vi "final_control_mk12_061625.vi"() -> ()   [LabVIEW 2023]
doc: "Simplified example program for initializing the COM port, determining the data frame of up to 26 Alicats, acquiring the data of the same number of Alicats, displaying the data of the one with the selected unit ID, and writing a setpoint to the same selected unit ID.\n\nThis is a slightly more feature rich version of the Alicat Simplified Driver Example, and contains an example of a method for interfacing with up to 26 Alicats on a single COM port by means of for loops with shift registers to handle sequential commands to each included Alicat. This also contains a method to write a setpoint to the same selected unit.\n\nIf coding for multiple Alicats on a single COM port without the use of for loops with shift registers, ensure that each Alicat command is executed sequentially. Alicat's RS-232/485 does not work if multiple devices are responding simultaneously."
uses:
  <vilib>/Platform/TimedLoop/XDataNode/timing_clust.ctl
  <vilib>/Platform/TimedLoop/XDataNode/nitl_modes.ctl
  <vilib>/Platform/TimedLoop/XDataNode/wakeup.ctl
  <vilib>/DAQmx/write.llb/DAQmx Write (Analog 1D DBL NChan 1Samp).vi
  <vilib>/DAQmx/read.llb/DAQmx Read (Analog DBL 1Chan 1Samp).vi
  <extravilib>/ChannelInstances/Tag-bool/Read With Abort.vi
  <extravilib>/ChannelInstances/Tag-bool/Write With Abort.vi
  <vilib>/Utility/file.llb/Write Delimited Spreadsheet (string).vi
  <extravilib>/ChannelInstances/Tag-bool/Instantiate.vi
  <vilib>/Utility/file.llb/Read Delimited Spreadsheet (DBL).vi
  <extravilib>/ChannelInstances/Tag-bool/EndpointRead.vi
  <vilib>/DAQmx/miscellaneous.llb/DAQmx Fill In Error Info.vi
  <extravilib>/ChannelInstances/Tag-bool/Endpoint.vi
  <vilib>/platform/TimedLoop/XDataNode/XDataNode.xnode
  <vilib>/express/express arith-compare/Formula/XNode/ExpressFormulaBlockNode.xnode
  <vilib>/Platform/TimedLoop/XDataNode/XDNodeRunTimeDep.lvlib
  <extravilib>/ChannelInstances/Tag-bool.lvlib
panel:
  in  "Tab Control":enum32{"Page 1", "Page 2"}(tab)
  in  "COM Port Settings":T1={"Baud Rate"=enum."19200", "VISA Sesssion In"="MassFlowControllers"}
  out "Range Exceeded":bool
  out "Error Present":bool
  out "Error Text":string
  out "Elapsed Time [ms]\n(all units)":dbl caption="Elapsed Time (s)"
  in  "Minimum time between \nreadings [ms] (all units)":u32
  in  "Device ID's \nto Include:":T2={"A"=TRUE, "B"=TRUE, "C"=TRUE, "D"=TRUE, "E"=TRUE, "F"=TRUE, "G"=FALSE, "H"=FALSE, "I"=FALSE, "J"=FALSE, "K"=FALSE, "L"=FALSE, "M"=FALSE, "N"=FALSE, "O"=FALSE, "P"=FALSE, "Q"=FALSE, "R"=FALSE, "S"=FALSE, "T"=FALSE, "U"=FALSE, "V"=FALSE, "W"=FALSE, "X"=FALSE, "Y"=FALSE, "Z"=FALSE}
  out "Active Device":u16(ring) items=["A", "B", "C", "D", "E", "F"]
  out "Meas. Data (for active device)":T3
  in  "Write File":path
  in  "Hold Time\n[min]":dbl=16.0 min=17.0
  out "N":i32
  in  "Read File":path
  in  "End Program":bool
  in  "Start From:":i32=1
  in  "t_read [ms]":dbl=24000.0
  out "T_SCh [C]":dbl format="%0.2f"
  out "iter start":string
  out "Iter_Duration [ms]":string
  out "C_CH4 [ppm]":string
  out "C_H2 [ppm]":string
  in  "Start Times":path
  in  "API Key":string="V1WFARF28XTM5DW7"
  in  "Send Alerts?":bool=TRUE
  out "C_H2S [ppm]":string
  out "len_SP":i32
  out "Setpoints":dbl[][](array[numeric])=[[4.2, 3.3], [69.0, 4.2]]
  out "Z":dbl[](array[numeric])
  out "ASP":dbl
  out "BSP":dbl
  out "CSP":dbl
  out "DSP":dbl
  out "ESP":dbl
  out "FSP":dbl
  out "N_read":i32
  out "Iter_#":string
  out "V_D":string
  out "V_H":string
  out "all rows":dbl[][](array[numeric])
  out "T_SCh":string
  out "Iteration Duration":i64
  out "read_cnt_true":i32
  out "iter_dur_read [ms]":i64
  out "t_diff":dbl
  out "date":string
  out "time":string
  # "Totalizer Timer"
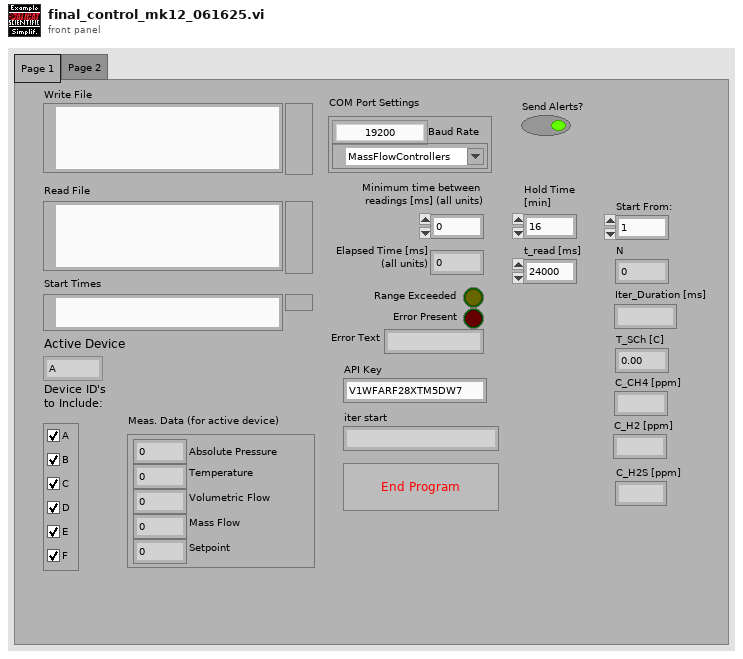
[diagram p1: front panel]
types:
  T1 = cluster{"Baud Rate":enum8{"2400", "9600", "19200", "38400", "57600", "115200", "Unknown"}, "VISA Sesssion In":refnum<visa-resource-name>}
  T2 = cluster{"A":bool, "B":bool, "C":bool, "D":bool, "E":bool, "F":bool, "G":bool, "H":bool, "I":bool, "J":bool, "K":bool, "L":bool, "M":bool, "N":bool, "O":bool, "P":bool, "Q":bool, "R":bool, "S":bool, "T":bool, "U":bool, "V":bool, "W":bool, "X":bool, "Y":bool, "Z":bool}
  T3 = cluster{"Absolute Pressure":dbl, "Gauge/Diff. Pressure":dbl, "Barometric Pressure":dbl, "Temperature":dbl, "Volumetric Flow":dbl, "Mass Flow":dbl, "Setpoint":dbl, "Valve Drive":dbl, "Totalizer":dbl, "[hr]":dbl, "[min]":dbl, "[sec]":dbl, "Totalizer Average Flow":dbl, "Totalizer Peak Flow":dbl, "Gas selected":string}
  T4 = cluster{"Unit ID":string, "Baud Rate":enum8{"2400", "9600", "19200", "38400", "57600", "115200", "Unknown"}, "VISA Sesssion In":refnum<visa-resource-name>}
  T5 = enum16{"Request Ack", "Set Setpoint", "Set Lo Limit", "Set Hi Limit", "Set Prop Band 0-99.9", "Set Integral 0-9.99", "Set Derivative 0-5.0", "Read Int Temp", "Read Ext Temp", "Read Setpoint", "Read Low Limit", "Read High Limit", "Read Prop Band", "Read Integral", "Read Derivative "}
  T6 = typedef "XDNodeRunTimeDep.lvlib/timing_clust.ctl" = cluster{"Expected End [f-1]":u64, "Actual End [f-1]":u64, "Finished Late? [f-1]":bool, "Expected End [i-1]":u64, "Actual End [i-1]":u64, "Finished Late? [i-1]":bool, "Expected Start [i]":u64, "Actual Start [i]":u64, "Expected Start [f]":u64, "Actual Start [f]":u64, "Source Name":string, "Structure Name":string, "Period":i64, "Deadline":i64, "Offset":i64, "Start":i64, "Priority":i32, "Timeout":i32, "Mode":T7, "Wakeup Reason":T8, "Error":errorcluster, "Source Type":string, "Secondary Source Type":string, "Global End Time":u64, "Global Start Time":u64, "Frame Duration":u64, "Iteration Duration":u64, "Assigned CPU":i32, "I/O Scan Engine Mode":u32}
  T7 = typedef "XDNodeRunTimeDep.lvlib/nitl_modes.ctl" = enum32{"No Change", "Process missed periods, maintain original phase", "Discard missed periods, maintain original phase", "Process missed periods, ignore original phase", "Discard missed periods, ignore original phase"}
  T8 = typedef "XDNodeRunTimeDep.lvlib/wakeup.ctl" = enum32{"Normal", "Aborted", "Asynchronous wakeup", "Timing source error", "Timed loop error", "Timeout"}
  T9 = typedef "Tag-bool.lvlib/))Channel.ctl" = refnum<queue>
  T10 = enum8{"2400", "9600", "19200", "38400", "57600", "115200", "Unknown"}
  T11 = cluster{"Absolute Pressure":bool, "Gauge/Diff. Pressure":bool, "Barometric Pressure":bool, "Temperature":bool, "Volumetric":bool, "Mass":bool, "Setpoint":bool, "Valve Drive":bool, "Totalizer":bool, "Totalizer Timer":bool, "Totalizer Average Flow":bool, "Totalizer Peak Flow":bool, "Gas Selected":bool, "Tot. Timer Format":u16}
  T12 = cluster{"Controller Full Scale":dbl, "Controller Select":u16, "Control Range":enum16{"Normal", "Inverted", "Bidirectional", "Unknown"}}
  T13 = cluster{"Controller Full Scale":dbl, "Controller Select":u16, "Control Range":enum16{"Normal", "Inverted", "Bidirectional", "Unknown"}}[]
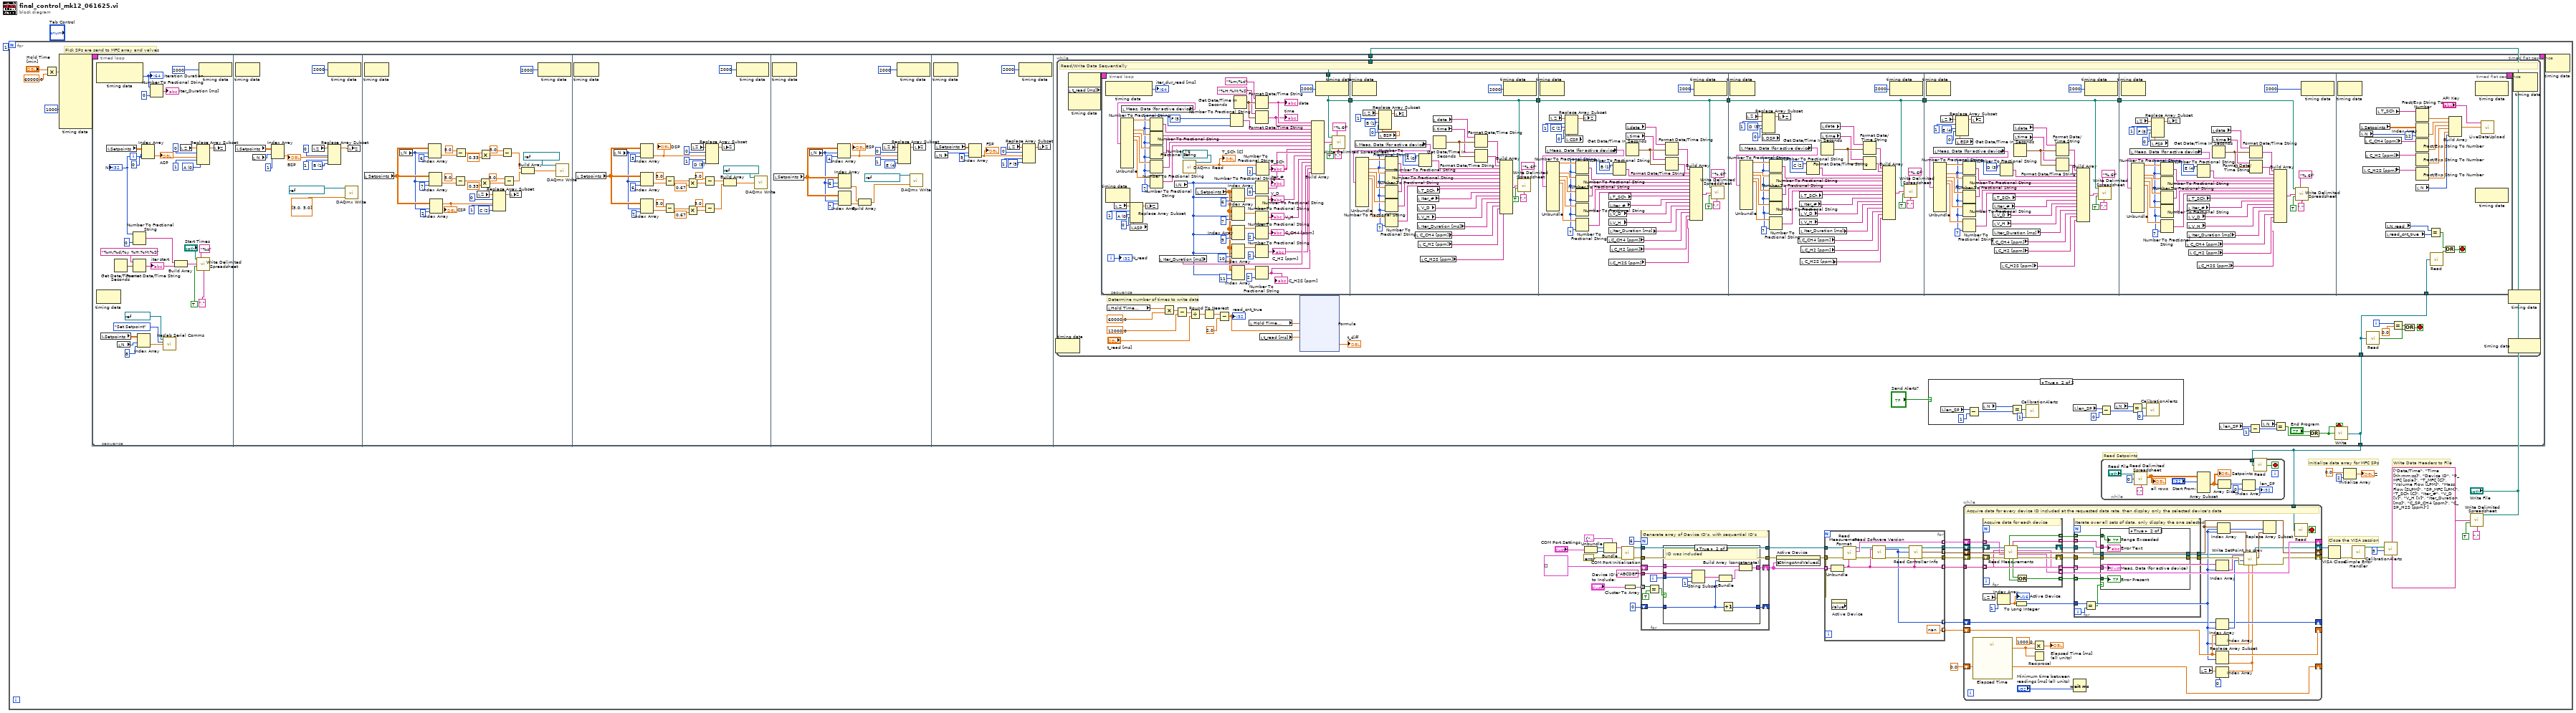
[diagram p0: block diagram]
diagram:
  n1 = for {
    N: 1 -> [_]
    # "Pick SPs are send to MFC array and valves"
    # "Write Data Headers to File"
    # "Read Setpoints"
    # "Initialize data array for MFC SPs"
    # "Close the VISA session"
    n2 = Multiply(x="Hold Time\n[min]", y=60000.0) -> (x*y=w5:dbl)
    n3 = node-c288(w5, i64 1000 ("Offset")) -> (w46:T6)  [unwired: 8 in]
    n4 = timed-loop "Write Data" {
      timing: w46 -> [_]
      timing-out: [_] -> w45
      tunnel: [w59] -> w12
      tunnel: "Write File" -> [w58]
      i -> [w73]
      stop <- w216 stop-if-true
      n5 = timed-sequence {
        timing: _ -> [_]
        timing-out: _ -> [_]
        tunnel: [w61] -> w59
        tunnel: w58 -> [w60]
        n6 = timed-flat-sequence {
          tunnel: [w211] -> w61
          tunnel: w60 -> [w212]
          frame #0 {
            w83 = u16 0 items=["A", "B", "C", "D", "E", "F"]
            n7 = node-c288() -> (w77:i64)  [unwired: 1 in, 1 out]
            "Iteration Duration" <- w77
            n8 = local read "Setpoints"() -> (w67:dbl[][])
            n9 = local read "Setpoints"() -> (w90:dbl[][])
            n10 = Get Date/Time In Seconds() -> (seconds since 1Jan1904=w78:timestamp)
            n11 = local read "N"() -> (w66:i32)
            n12 = Number To Fractional String(number=w73, precision (6)=i16 0) -> (F-format string=w71:string)  [unwired: 2 in]
            n13 = Format Date/Time String(time format string (%c)="%m/%d/%y %H:%M:%S", seconds (now)=w78) -> (date/time string=w70:string)  [unwired: 1 in]
            "iter start" <- w70
            n14 = Index Array(array=w67, index (row)=w66, index (col)=8 ("disabled index (col)")) -> (element=w64:dbl)
            n15 = Index Array(array=w90, index (row)=w73, index (col)=0 ("index (row)")) -> (element=w88:dbl)
            "ASP" <- w88
            n16 = Number To Fractional String(number=w77, precision (6)=i16 0) -> (F-format string=→"Iter_Duration [ms]":string)  [unwired: 2 in]
            n17 = call "Neslab Serial Comms.vi"("VISA resource name"=refnum<visa-resource-name> "COM1", "Command"=T5."Set Setpoint", "Set Value"=w64) -> ()  [unwired: 6 in, 7 out]
            n18 = Build Array(w71, w70) -> (w69:string[])
            n19 = local read "Z"() -> (w86:dbl[])
            n20 = Replace Array Subset(array=w86, new element #1=w88, index #1=0 ("index"), new element #2=w83, index #2=1 ("index")) -> (w87:dbl[])
            n21 = call-poly <vilib>:"Write Delimited Spreadsheet.vi"("file path (dialog if empty)"="Start Times", "format (%s)"="%s" ("format (%.3f)"), "1D data"=w69, "append to file? (new file:F)"=TRUE, "delimiter (\\t)"="," ("delimiter (\\t)")) -> ()  [unwired: 9 in, 2 out]
            n22 = node-c288(i64 2000 ("Start")) -> ()  [unwired: 1 out]
            n23 = local write "Z"(w87) -> ()
            "N" <- w73
          }
          frame #1 {
            w98 = u16 1 items=["A", "B", "C", "D", "E", "F"]
            n24 = node-c288() -> ()  [unwired: 1 in, 1 out]
            n25 = local read "Setpoints"() -> (w106:dbl[][])
            n26 = local read "N"() -> (w99:i32)
            n27 = Index Array(array=w106, index (row)=w99, index (col)=1 ("index (row)")) -> (element=w103:dbl)
            "BSP" <- w103
            n28 = local read "Z"() -> (w101:dbl[])
            n29 = Replace Array Subset(array=w101, new element #1=w103, index #1=0 ("index"), new element #2=w98, index #2=1 ("index")) -> (w102:dbl[])
            n30 = node-c288(i64 2000 ("Start")) -> ()  [unwired: 1 out]
            n31 = call-poly <vilib>:"DAQmx Write.vi"("task/channels in"=refnum<k21> "Valve_cont", "data"=dbl[] [5.0, 5.0]) -> ()  [unwired: 11 in, 3 out]
            n32 = local write "Z"(w102) -> ()
          }
          frame #2 {
            w113 = u16 2 items=["A", "B", "C", "D", "E", "F"]
            n33 = node-c288() -> ()  [unwired: 1 in, 1 out]
            n34 = local read "Setpoints"() -> (w125:dbl[][])
            n35 = local read "N"() -> (w124:i32)
            n36 = Index Array(array=w125, index (row)=w124, index (col)=6 ("disabled index (col)")) -> (element=w115:dbl)
            n37 = Index Array(array=w125, index (row)=w124, index (col)=7 ("disabled index (col)")) -> (element=w123:dbl)
            n38 = Index Array(array=w125, index (row)=w124, index (col)=2 ("index (row)")) -> (element=w137:dbl)
            "CSP" <- w137
            n39 = Subtract(x=5.0, y=w123) -> (x-y=w132:dbl)
            n40 = Subtract(x=5.0, y=w115) -> (x-y=w119:dbl)
            n41 = local read "Z"() -> (w135:dbl[])
            n42 = Multiply(x=w132, y=0.33) -> (x*y=w130:dbl)
            n43 = Multiply(x=w119, y=0.33) -> (x*y=w117:dbl)
            n44 = Replace Array Subset(array=w135, new element #1=w137, index #1=0 ("index"), new element #2=w113, index #2=1 ("index")) -> (w136:dbl[])
            n45 = Subtract(x=5.0, y=w117) -> (x-y=w114:dbl)
            n46 = Subtract(x=5.0, y=w130) -> (x-y=w127:dbl)
            n47 = local write "Z"(w136) -> ()
            n48 = Build Array(w114, w127) -> (w126:dbl[])
            n49 = node-c288(i64 2000 ("Start")) -> ()  [unwired: 1 out]
            n50 = call-poly <vilib>:"DAQmx Write.vi"("task/channels in"=refnum<k21> "Valve_cont", "data"=w126) -> ()  [unwired: 11 in, 3 out]
          }
          frame #3 {
            w164 = u16 3 items=["A", "B", "C", "D", "E", "F"]
            n51 = node-c288() -> ()  [unwired: 1 in, 1 out]
            n52 = local read "Setpoints"() -> (w153:dbl[][])
            n53 = local read "N"() -> (w152:i32)
            n54 = Index Array(array=w153, index (row)=w152, index (col)=7 ("disabled index (col)")) -> (element=w145:dbl)
            n55 = Index Array(array=w153, index (row)=w152, index (col)=3 ("index (row)")) -> (element=w168:dbl)
            "DSP" <- w168
            n56 = Index Array(array=w153, index (row)=w152, index (col)=6 ("disabled index (col)")) -> (element=w151:dbl)
            n57 = Subtract(x=5.0, y=w151) -> (x-y=w161:dbl)
            n58 = Subtract(x=5.0, y=w145) -> (x-y=w149:dbl)
            n59 = Multiply(x=w161, y=0.67) -> (x*y=w159:dbl)
            n60 = Multiply(x=w149, y=0.67) -> (x*y=w147:dbl)
            n61 = local read "Z"() -> (w166:dbl[])
            n62 = Subtract(x=5.0, y=w159) -> (x-y=w155:dbl)
            n63 = Subtract(x=5.0, y=w147) -> (x-y=w144:dbl)
            n64 = Replace Array Subset(array=w166, new element #1=w168, index #1=0 ("index"), new element #2=w164, index #2=1 ("index")) -> (w167:dbl[])
            n65 = local write "Z"(w167) -> ()
            n66 = Build Array(w155, w144) -> (w154:dbl[])
            n67 = node-c288(i64 2000 ("Start")) -> ()  [unwired: 1 out]
            n68 = call-poly <vilib>:"DAQmx Write.vi"("task/channels in"=refnum<k21> "Valve_cont", "data"=w154) -> ()  [unwired: 11 in, 3 out]
          }
          frame #4 {
            w185 = u16 4 items=["A", "B", "C", "D", "E", "F"]
            n69 = node-c288() -> ()  [unwired: 1 in, 1 out]
            n70 = local read "Setpoints"() -> (w180:dbl[][])
            n71 = local read "N"() -> (w179:i32)
            n72 = Index Array(array=w180, index (row)=w179, index (col)=4 ("index (row)")) -> (element=w189:dbl)
            "ESP" <- w189
            n73 = Index Array(array=w180, index (row)=w179, index (col)=6 ("disabled index (col)")) -> (element=w182:dbl)
            n74 = Index Array(array=w180, index (row)=w179, index (col)=7 ("disabled index (col)")) -> (element=w181:dbl)
            n75 = Build Array(w182, w181) -> (w178:dbl[])
            n76 = local read "Z"() -> (w187:dbl[])
            n77 = node-c288(i64 2000 ("Start")) -> ()  [unwired: 1 out]
            n78 = Replace Array Subset(array=w187, new element #1=w189, index #1=0 ("index"), new element #2=w185, index #2=1 ("index")) -> (w188:dbl[])
            n79 = call-poly <vilib>:"DAQmx Write.vi"("task/channels in"=refnum<k21> "Valve_cont", "data"=w178) -> ()  [unwired: 11 in, 3 out]
            n80 = local write "Z"(w188) -> ()
          }
          frame #5 {
            w199 = u16 5 items=["A", "B", "C", "D", "E", "F"]
            n81 = node-c288() -> ()  [unwired: 1 in, 1 out]
            n82 = local read "Setpoints"() -> (w202:dbl[][])
            n83 = local read "N"() -> (w197:i32)
            n84 = Index Array(array=w202, index (row)=w197, index (col)=5 ("index (row)")) -> (element=w198:dbl)
            "FSP" <- w198
            n85 = local read "Z"() -> (w201:dbl[])
            n86 = node-c288(i64 2000 ("Start")) -> ()  [unwired: 1 out]
            n87 = Replace Array Subset(array=w201, new element #1=w198, index #1=0 ("index"), new element #2=w199, index #2=1 ("index")) -> (w200:dbl[])
            n88 = local write "Z"(w200) -> ()
          }
          frame #6 {
            n89 = node-c288() -> ()  [unwired: 1 in, 1 out]
            n90 = case shown="True" "Send Alerts?" {
              frame False {
              }
              frame True {
                n91 = local read "len_SP"() -> (w223:i32)
                n92 = Subtract(x=w223, y=1) -> (x-y=w225:i32)
                n93 = local read "N"() -> (w224:i32)
                n94 = Equal?(x=w224, y=w225) -> (x = y?=w221:bool)
                n95 = call "CalibrationAlerts.vi"("Alert Type (0)"=1, "Trigger"=w221) -> ()  [unwired: 10 in]
                n96 = local read "len_SP"() -> (w228:i32)
                n97 = Subtract(x=w228, y=0) -> (x-y=w227:i32)
                n98 = local read "N"() -> (w231:i32)
                n99 = Equal?(x=w231, y=w227) -> (x = y?=w220:bool)
                n100 = call "CalibrationAlerts.vi"("Alert Type (0)"=0, "Trigger"=w220) -> ()  [unwired: 10 in]
              }
            }
            n101 = local read "len_SP"() -> (w215:i32)
            n102 = Subtract(x=w215, y=1) -> (x-y=w218:i32)
            n103 = local read "N"() -> (w214:i32)
            n104 = Equal?(x=w214, y=w218) -> (x = y?=w217:bool)
            n105 = Or(x="End Program", y=w217) -> (x .or. y?=w216:bool)
            n106 = call <extravilib>:"Write.vi"("element"=w216) -> ("channel"=w211:T9)  [unwired: 1 out]
            n107 = while {
              tunnel: w212 -> [w252]
              tunnel: w211 -> [w242]
              i -> [w241]
              stop <- w248 stop-if-true
              # "Determine number of times to write data"
              # "Read/Write Data Sequentially"
              n108 = local read "t_read [ms]"() -> (w232:dbl)
              n109 = node-c288(w232) -> (w254:T6)  [unwired: 3 in]
              n110 = timed-loop {
                timing: w254 -> [_]
                timing-out: [_] -> w253
                tunnel: w252 -> [w267]
                tunnel: w242 -> [w268]
                i -> [w335]
                stop <- w574 stop-if-true
                n111 = timed-sequence {
                  timing: _ -> [_]
                  timing-out: _ -> [_]
                  tunnel: w268 -> [w270]
                  tunnel: w267 -> [w269]
                  n112 = timed-flat-sequence {
                    tunnel: [w301] -> w275
                    tunnel: w269 -> [w301]
                    tunnel: w275 -> [w367]
                    tunnel: [w367] -> w274
                    tunnel: w274 -> [w403]
                    tunnel: [w403] -> w273
                    tunnel: w273 -> [w442]
                    tunnel: [w442] -> w272
                    tunnel: w272 -> [w475]
                    tunnel: [w475] -> w271
                    tunnel: w271 -> [w529]
                    tunnel: w270 -> [w573]
                    frame #0 {
                      w316 = u16 5 items=["A", "B", "C", "D", "E", "F"]
                      w319 = u16 0 items=["A", "B", "C", "D", "E", "F"]
                      w312 = i16 7 ("precision (6)")
                      n113 = node-c288() -> (→"iter_dur_read [ms]":i64)  [unwired: 1 in]
                      n114 = local read "Z"() -> (w305:dbl[])
                      n115 = local read "Meas. Data (for active device)"() -> (w302:T3)
                      n116 = Unbundle(w302) -> ("Absolute Pressure"=w325:dbl, "Temperature"=w315:dbl, "Volumetric Flow"=w321:dbl, "Mass Flow"=w314:dbl, "Setpoint"=w313:dbl)  [unwired: 10 out]
                      n117 = local read "ASP"() -> (w303:dbl)
                      n118 = Replace Array Subset(array=w305, new element #1=w319, index #1=1 ("index"), new element #2=w303, index #2=0 ("index")) -> (w304:dbl[])
                      n119 = local write "Z"(w304) -> ()
                      n120 = Number To Fractional String(number=w325, precision (6)=w312) -> (F-format string=w310:string)  [unwired: 2 in]
                      n121 = Number To Fractional String(number=w315, precision (6)=w312) -> (F-format string=w308:string)  [unwired: 2 in]
                      n122 = Number To Fractional String(number=w321, precision (6)=w312) -> (F-format string=w309:string)  [unwired: 2 in]
                      n123 = Number To Fractional String(number=w314, precision (6)=w312) -> (F-format string=w307:string)  [unwired: 2 in]
                      n124 = Number To Fractional String(number=w313, precision (6)=w312) -> (F-format string=w306:string)  [unwired: 2 in]
                      n125 = local read "Iter_Duration [ms]"() -> (w300:string)
                      n126 = local read "N"() -> (w277:i32)
                      n127 = call-poly <vilib>:"DAQmx Read.vi"("task/channels in"=refnum<k21> "Temp") -> ("data"=w328:dbl)  [unwired: 12 in, 2 out]
                      "T_SCh [C]" <- w328
                      n128 = local read "Setpoints"() -> (w279:dbl[][])
                      n129 = Number To Fractional String(number=w316, precision (6)=w312) -> (F-format string=w311:string)  [unwired: 2 in]
                      n130 = Index Array(array=w279, index (row)=w277, index (col)=6 ("disabled index (col)")) -> (element=w332:dbl)
                      n131 = Index Array(array=w279, index (row)=w277, index (col)=7 ("disabled index (col)")) -> (element=w331:dbl)
                      n132 = Index Array(array=w279, index (row)=w277, index (col)=9 ("disabled index (col)")) -> (element=w288:dbl)
                      n133 = Index Array(array=w279, index (row)=w277, index (col)=10 ("disabled index (col)")) -> (element=w284:dbl)
                      n134 = Index Array(array=w279, index (row)=w277, index (col)=11) -> (element=w278:dbl)
                      n135 = Get Date/Time In Seconds() -> (seconds since 1Jan1904=w294:timestamp)
                      n136 = Format Date/Time String(time format string (%c)="%m/%d", seconds (now)=w294) -> (date/time string=w296:string)  [unwired: 1 in]
                      "date" <- w296
                      n137 = Format Date/Time String(time format string (%c)="%H:%M:%S", seconds (now)=w294) -> (date/time string=w295:string)  [unwired: 1 in]
                      "time" <- w295
                      n138 = Number To Fractional String(number=w277, precision (6)=i16 0) -> (F-format string=w297:string)  [unwired: 2 in]
                      "Iter_#" <- w297
                      n139 = Number To Fractional String(number=w332) -> (F-format string=w298:string)  [unwired: 3 in]
                      "V_D" <- w298
                      n140 = Number To Fractional String(number=w331) -> (F-format string=w299:string)  [unwired: 3 in]
                      "V_H" <- w299
                      n141 = Number To Fractional String(number=w288, precision (6)=i16 2) -> (F-format string=w286:string)  [unwired: 2 in]
                      "C_CH4 [ppm]" <- w286
                      n142 = Number To Fractional String(number=w284, precision (6)=i16 2) -> (F-format string=w282:string)  [unwired: 2 in]
                      "C_H2 [ppm]" <- w282
                      n143 = Number To Fractional String(number=w278, precision (6)=i16 2) -> (F-format string=w276:string)  [unwired: 2 in]
                      "C_H2S [ppm]" <- w276
                      n144 = Number To Fractional String(number=w328, precision (6)=i16 2) -> (F-format string=w291:string)  [unwired: 2 in]
                      "T_SCh" <- w291
                      n145 = Build Array(w296, w295, w311, w310, w308, w309, w307, w306, w291, w297, w298, w299, w300, w286, w282, w276) -> (w322:string[])
                      n146 = node-c288(i64 2000 ("Start")) -> ()  [unwired: 1 out]
                      n147 = call-poly <vilib>:"Write Delimited Spreadsheet.vi"("file path (dialog if empty)"=w301, "format (%s)"="%.6f" ("format (%.3f)"), "1D data"=w322, "append to file? (new file:F)"=TRUE, "delimiter (\\t)"="," ("delimiter (\\t)")) -> ()  [unwired: 9 in, 2 out]
                      "N_read" <- w335
                    }
                    frame #1 {
                      w364 = u16 0 items=["A", "B", "C", "D", "E", "F"]
                      w373 = u16 1 items=["A", "B", "C", "D", "E", "F"]
                      w360 = i16 7 ("precision (6)")
                      n148 = node-c288() -> ()  [unwired: 1 in, 1 out]
                      n149 = local read "Meas. Data (for active device)"() -> (w371:T3)
                      n150 = Unbundle(w371) -> ("Absolute Pressure"=w379:dbl, "Temperature"=w363:dbl, "Volumetric Flow"=w375:dbl, "Mass Flow"=w362:dbl, "Setpoint"=w361:dbl)  [unwired: 10 out]
                      n151 = local read "Z"() -> (w370:dbl[])
                      n152 = local read "BSP"() -> (w365:dbl)
                      n153 = Replace Array Subset(array=w370, new element #1=w373, index #1=1 ("index"), new element #2=w365, index #2=0 ("index")) -> (w369:dbl[])
                      n154 = Number To Fractional String(number=w379, precision (6)=w360) -> (F-format string=w358:string)  [unwired: 2 in]
                      n155 = Number To Fractional String(number=w363, precision (6)=w360) -> (F-format string=w356:string)  [unwired: 2 in]
                      n156 = Number To Fractional String(number=w375, precision (6)=w360) -> (F-format string=w357:string)  [unwired: 2 in]
                      n157 = Number To Fractional String(number=w362, precision (6)=w360) -> (F-format string=w355:string)  [unwired: 2 in]
                      n158 = Number To Fractional String(number=w361, precision (6)=w360) -> (F-format string=w354:string)  [unwired: 2 in]
                      n159 = local write "Z"(w369) -> ()
                      n160 = local read "C_CH4 [ppm]"() -> (w343:string)
                      n161 = local read "T_SCh"() -> (w353:string)
                      n162 = local read "Iter_#"() -> (w352:string)
                      n163 = local read "V_D"() -> (w351:string)
                      n164 = local read "V_H"() -> (w350:string)
                      n165 = local read "Iter_Duration [ms]"() -> (w349:string)
                      n166 = local read "C_H2 [ppm]"() -> (w342:string)
                      n167 = Number To Fractional String(number=w364, precision (6)=w360) -> (F-format string=w359:string)  [unwired: 2 in]
                      n168 = local read "C_H2S [ppm]"() -> (w341:string)
                      n169 = local read "date"() -> (w344:string)
                      n170 = local read "time"() -> (w345:string)
                      n171 = Get Date/Time In Seconds() -> (seconds since 1Jan1904=w346:timestamp)
                      n172 = Format Date/Time String(time format string (%c)=w344, seconds (now)=w346) -> (date/time string=w348:string)  [unwired: 1 in]
                      n173 = Format Date/Time String(time format string (%c)=w345, seconds (now)=w346) -> (date/time string=w347:string)  [unwired: 1 in]
                      n174 = Build Array(w348, w347, w359, w358, w356, w357, w355, w354, w353, w352, w351, w350, w349, w343, w342, w341) -> (w376:string[])
                      n175 = node-c288(i64 2000 ("Start")) -> ()  [unwired: 1 out]
                      n176 = call-poly <vilib>:"Write Delimited Spreadsheet.vi"("file path (dialog if empty)"=w367, "format (%s)"="%.6f" ("format (%.3f)"), "1D data"=w376, "append to file? (new file:F)"=TRUE, "delimiter (\\t)"="," ("delimiter (\\t)")) -> ()  [unwired: 9 in, 2 out]
                    }
                    frame #2 {
                      w409 = u16 1 items=["A", "B", "C", "D", "E", "F"]
                      w408 = i16 7 ("precision (6)")
                      w421 = u16 2 items=["A", "B", "C", "D", "E", "F"]
                      n177 = node-c288() -> ()  [unwired: 1 in, 1 out]
                      n178 = local read "Meas. Data (for active device)"() -> (w410:T3)
                      n179 = Unbundle(w410) -> ("Absolute Pressure"=w415:dbl, "Temperature"=w413:dbl, "Volumetric Flow"=w414:dbl, "Mass Flow"=w412:dbl, "Setpoint"=w411:dbl)  [unwired: 10 out]
                      n180 = local read "Z"() -> (w420:dbl[])
                      n181 = local read "CSP"() -> (w416:dbl)
                      n182 = Replace Array Subset(array=w420, new element #1=w421, index #1=1 ("index"), new element #2=w416, index #2=0 ("index")) -> (w419:dbl[])
                      n183 = Number To Fractional String(number=w415, precision (6)=w408) -> (F-format string=w396:string)  [unwired: 2 in]
                      n184 = Number To Fractional String(number=w413, precision (6)=w408) -> (F-format string=w395:string)  [unwired: 2 in]
                      n185 = Number To Fractional String(number=w414, precision (6)=w408) -> (F-format string=w394:string)  [unwired: 2 in]
                      n186 = Number To Fractional String(number=w412, precision (6)=w408) -> (F-format string=w393:string)  [unwired: 2 in]
                      n187 = Number To Fractional String(number=w411, precision (6)=w408) -> (F-format string=w392:string)  [unwired: 2 in]
                      n188 = local write "Z"(w419) -> ()
                      n189 = local read "C_CH4 [ppm]"() -> (w386:string)
                      n190 = local read "T_SCh"() -> (w402:string)
                      n191 = local read "Iter_#"() -> (w401:string)
                      n192 = local read "V_D"() -> (w400:string)
                      n193 = local read "V_H"() -> (w399:string)
                      n194 = local read "Iter_Duration [ms]"() -> (w398:string)
                      n195 = local read "C_H2S [ppm]"() -> (w384:string)
                      n196 = local read "C_H2 [ppm]"() -> (w385:string)
                      n197 = Number To Fractional String(number=w409, precision (6)=w408) -> (F-format string=w397:string)  [unwired: 2 in]
                      n198 = local read "date"() -> (w387:string)
                      n199 = local read "time"() -> (w388:string)
                      n200 = Get Date/Time In Seconds() -> (seconds since 1Jan1904=w389:timestamp)
                      n201 = Format Date/Time String(time format string (%c)=w387, seconds (now)=w389) -> (date/time string=w391:string)  [unwired: 1 in]
                      n202 = Format Date/Time String(time format string (%c)=w388, seconds (now)=w389) -> (date/time string=w390:string)  [unwired: 1 in]
                      n203 = Build Array(w391, w390, w397, w396, w395, w394, w393, w392, w402, w401, w400, w399, w398, w386, w385, w384) -> (w404:string[])
                      n204 = node-c288(i64 2000 ("Start")) -> ()  [unwired: 1 out]
                      n205 = call-poly <vilib>:"Write Delimited Spreadsheet.vi"("file path (dialog if empty)"=w403, "format (%s)"="%.6f" ("format (%.3f)"), "1D data"=w404, "append to file? (new file:F)"=TRUE, "delimiter (\\t)"="," ("delimiter (\\t)")) -> ()  [unwired: 9 in, 2 out]
                    }
                    frame #3 {
                      w436 = u16 3 items=["A", "B", "C", "D", "E", "F"]
                      w459 = u16 2 items=["A", "B", "C", "D", "E", "F"]
                      w458 = i16 7 ("precision (6)")
                      n206 = node-c288() -> ()  [unwired: 1 in, 1 out]
                      n207 = local read "Meas. Data (for active device)"() -> (w441:T3)
                      n208 = Unbundle(w441) -> ("Absolute Pressure"=w464:dbl, "Temperature"=w462:dbl, "Volumetric Flow"=w463:dbl, "Mass Flow"=w461:dbl, "Setpoint"=w460:dbl)  [unwired: 10 out]
                      n209 = local read "Z"() -> (w439:dbl[])
                      n210 = local read "DSP"() -> (w440:dbl)
                      n211 = Replace Array Subset(array=w439, new element #1=w436, index #1=1 ("index"), new element #2=w440, index #2=0 ("index")) -> (w438:dbl[])
                      n212 = Number To Fractional String(number=w464, precision (6)=w458) -> (F-format string=w452:string)  [unwired: 2 in]
                      n213 = Number To Fractional String(number=w462, precision (6)=w458) -> (F-format string=w451:string)  [unwired: 2 in]
                      n214 = Number To Fractional String(number=w463, precision (6)=w458) -> (F-format string=w450:string)  [unwired: 2 in]
                      n215 = Number To Fractional String(number=w461, precision (6)=w458) -> (F-format string=w449:string)  [unwired: 2 in]
                      n216 = Number To Fractional String(number=w460, precision (6)=w458) -> (F-format string=w448:string)  [unwired: 2 in]
                      n217 = local write "Z"(w438) -> ()
                      n218 = local read "C_CH4 [ppm]"() -> (w429:string)
                      n219 = local read "T_SCh"() -> (w443:string)
                      n220 = local read "Iter_#"() -> (w444:string)
                      n221 = local read "V_D"() -> (w445:string)
                      n222 = local read "V_H"() -> (w446:string)
                      n223 = local read "Iter_Duration [ms]"() -> (w447:string)
                      n224 = local read "C_H2S [ppm]"() -> (w427:string)
                      n225 = local read "C_H2 [ppm]"() -> (w428:string)
                      n226 = Number To Fractional String(number=w459, precision (6)=w458) -> (F-format string=w453:string)  [unwired: 2 in]
                      n227 = local read "date"() -> (w430:string)
                      n228 = local read "time"() -> (w431:string)
                      n229 = Get Date/Time In Seconds() -> (seconds since 1Jan1904=w432:timestamp)
                      n230 = Format Date/Time String(time format string (%c)=w430, seconds (now)=w432) -> (date/time string=w434:string)  [unwired: 1 in]
                      n231 = Format Date/Time String(time format string (%c)=w431, seconds (now)=w432) -> (date/time string=w433:string)  [unwired: 1 in]
                      n232 = Build Array(w434, w433, w453, w452, w451, w450, w449, w448, w443, w444, w445, w446, w447, w429, w428, w427) -> (w454:string[])
                      n233 = node-c288(i64 2000 ("Start")) -> ()  [unwired: 1 out]
                      n234 = call-poly <vilib>:"Write Delimited Spreadsheet.vi"("file path (dialog if empty)"=w442, "format (%s)"="%.6f" ("format (%.3f)"), "1D data"=w454, "append to file? (new file:F)"=TRUE, "delimiter (\\t)"="," ("delimiter (\\t)")) -> ()  [unwired: 9 in, 2 out]
                    }
                    frame #4 {
                      w483 = u16 4 items=["A", "B", "C", "D", "E", "F"]
                      w502 = u16 3 items=["A", "B", "C", "D", "E", "F"]
                      w501 = i16 7 ("precision (6)")
                      n235 = node-c288() -> ()  [unwired: 1 in, 1 out]
                      n236 = local read "Meas. Data (for active device)"() -> (w485:T3)
                      n237 = Unbundle(w485) -> ("Absolute Pressure"=w507:dbl, "Temperature"=w505:dbl, "Volumetric Flow"=w506:dbl, "Mass Flow"=w504:dbl, "Setpoint"=w503:dbl)  [unwired: 10 out]
                      n238 = local read "Z"() -> (w480:dbl[])
                      n239 = local read "ESP"() -> (w481:dbl)
                      n240 = Replace Array Subset(array=w480, new element #1=w483, index #1=1 ("index"), new element #2=w481, index #2=0 ("index")) -> (w479:dbl[])
                      n241 = Number To Fractional String(number=w507, precision (6)=w501) -> (F-format string=w495:string)  [unwired: 2 in]
                      n242 = Number To Fractional String(number=w505, precision (6)=w501) -> (F-format string=w494:string)  [unwired: 2 in]
                      n243 = Number To Fractional String(number=w506, precision (6)=w501) -> (F-format string=w493:string)  [unwired: 2 in]
                      n244 = Number To Fractional String(number=w504, precision (6)=w501) -> (F-format string=w492:string)  [unwired: 2 in]
                      n245 = Number To Fractional String(number=w503, precision (6)=w501) -> (F-format string=w491:string)  [unwired: 2 in]
                      n246 = local write "Z"(w479) -> ()
                      n247 = local read "C_CH4 [ppm]"() -> (w472:string)
                      n248 = local read "T_SCh"() -> (w490:string)
                      n249 = local read "Iter_#"() -> (w486:string)
                      n250 = local read "V_D"() -> (w487:string)
                      n251 = local read "V_H"() -> (w488:string)
                      n252 = local read "Iter_Duration [ms]"() -> (w489:string)
                      n253 = local read "C_H2 [ppm]"() -> (w471:string)
                      n254 = Number To Fractional String(number=w502, precision (6)=w501) -> (F-format string=w496:string)  [unwired: 2 in]
                      n255 = local read "C_H2S [ppm]"() -> (w470:string)
                      n256 = local read "date"() -> (w473:string)
                      n257 = local read "time"() -> (w474:string)
                      n258 = Get Date/Time In Seconds() -> (seconds since 1Jan1904=w476:timestamp)
                      n259 = Format Date/Time String(time format string (%c)=w473, seconds (now)=w476) -> (date/time string=w478:string)  [unwired: 1 in]
                      n260 = Format Date/Time String(time format string (%c)=w474, seconds (now)=w476) -> (date/time string=w477:string)  [unwired: 1 in]
                      n261 = Build Array(w478, w477, w496, w495, w494, w493, w492, w491, w490, w486, w487, w488, w489, w472, w471, w470) -> (w497:string[])
                      n262 = node-c288(i64 2000 ("Start")) -> ()  [unwired: 1 out]
                      n263 = call-poly <vilib>:"Write Delimited Spreadsheet.vi"("file path (dialog if empty)"=w475, "format (%s)"="%.6f" ("format (%.3f)"), "1D data"=w497, "append to file? (new file:F)"=TRUE, "delimiter (\\t)"="," ("delimiter (\\t)")) -> ()  [unwired: 9 in, 2 out]
                    }
                    frame #5 {
                      w527 = u16 5 items=["A", "B", "C", "D", "E", "F"]
                      w546 = u16 4 items=["A", "B", "C", "D", "E", "F"]
                      w545 = i16 7 ("precision (6)")
                      n264 = node-c288() -> ()  [unwired: 1 in, 1 out]
                      n265 = local read "Meas. Data (for active device)"() -> (w530:T3)
                      n266 = Unbundle(w530) -> ("Absolute Pressure"=w551:dbl, "Temperature"=w549:dbl, "Volumetric Flow"=w550:dbl, "Mass Flow"=w548:dbl, "Setpoint"=w547:dbl)  [unwired: 10 out]
                      n267 = local read "Z"() -> (w523:dbl[])
                      n268 = local read "FSP"() -> (w525:dbl)
                      n269 = Replace Array Subset(array=w523, new element #1=w527, index #1=1 ("index"), new element #2=w525, index #2=0 ("index")) -> (w524:dbl[])
                      n270 = Number To Fractional String(number=w551, precision (6)=w545) -> (F-format string=w539:string)  [unwired: 2 in]
                      n271 = Number To Fractional String(number=w549, precision (6)=w545) -> (F-format string=w538:string)  [unwired: 2 in]
                      n272 = Number To Fractional String(number=w550, precision (6)=w545) -> (F-format string=w537:string)  [unwired: 2 in]
                      n273 = Number To Fractional String(number=w548, precision (6)=w545) -> (F-format string=w536:string)  [unwired: 2 in]
                      n274 = Number To Fractional String(number=w547, precision (6)=w545) -> (F-format string=w535:string)  [unwired: 2 in]
                      n275 = local write "Z"(w524) -> ()
                      n276 = local read "C_CH4 [ppm]"() -> (w517:string)
                      n277 = local read "T_SCh"() -> (w514:string)
                      n278 = local read "Iter_#"() -> (w531:string)
                      n279 = local read "V_D"() -> (w532:string)
                      n280 = local read "V_H"() -> (w533:string)
                      n281 = local read "Iter_Duration [ms]"() -> (w534:string)
                      n282 = local read "C_H2 [ppm]"() -> (w516:string)
                      n283 = local read "C_H2S [ppm]"() -> (w513:string)
                      n284 = Number To Fractional String(number=w546, precision (6)=w545) -> (F-format string=w540:string)  [unwired: 2 in]
                      n285 = local read "date"() -> (w518:string)
                      n286 = local read "time"() -> (w519:string)
                      n287 = Get Date/Time In Seconds() -> (seconds since 1Jan1904=w520:timestamp)
                      n288 = Format Date/Time String(time format string (%c)=w518, seconds (now)=w520) -> (date/time string=w522:string)  [unwired: 1 in]
                      n289 = Format Date/Time String(time format string (%c)=w519, seconds (now)=w520) -> (date/time string=w521:string)  [unwired: 1 in]
                      n290 = Build Array(w522, w521, w540, w539, w538, w537, w536, w535, w514, w531, w532, w533, w534, w517, w516, w513) -> (w541:string[])
                      n291 = call-poly <vilib>:"Write Delimited Spreadsheet.vi"("file path (dialog if empty)"=w529, "format (%s)"="%.6f" ("format (%.3f)"), "1D data"=w541, "append to file? (new file:F)"=TRUE, "delimiter (\\t)"="," ("delimiter (\\t)")) -> ()  [unwired: 9 in, 2 out]
                      n292 = node-c288(i64 2000 ("Start")) -> ()  [unwired: 1 out]
                    }
                    frame #6 {
                      n293 = node-c288() -> ()  [unwired: 1 in, 1 out]
                      n294 = local read "Setpoints"() -> (w565:dbl[][])
                      n295 = local read "N"() -> (w564:i32)
                      n296 = local read "C_H2S [ppm]"() -> (w557:string)
                      n297 = local read "C_CH4 [ppm]"() -> (w567:string)
                      n298 = local read "C_H2 [ppm]"() -> (w566:string)
                      n299 = local read "T_SCh"() -> (w569:string)
                      n300 = local read "N_read"() -> (w571:i32)
                      n301 = local read "read_cnt_true"() -> (w572:i32)
                      n302 = Fract/Exp String To Number(string=w569) -> (number=w568:dbl)  [unwired: 3 in, 1 out]
                      n303 = Index Array(array=w565, index (row)=w564, index (col)=12 ("disabled index (col)")) -> (element=w562:dbl)
                      n304 = Fract/Exp String To Number(string=w567) -> (number=w561:dbl)  [unwired: 3 in, 1 out]
                      n305 = Fract/Exp String To Number(string=w566) -> (number=w560:dbl)  [unwired: 3 in, 1 out]
                      n306 = Fract/Exp String To Number(string=w557) -> (number=w556:dbl)  [unwired: 3 in, 1 out]
                      n307 = local read "N"() -> (w559:i32)
                      n308 = Equal?(x=w571, y=w572) -> (x = y?=w576:bool)
                      n309 = call <extravilib>:"Read.vi"("channel"=w573) -> ("element"=w575:bool)  [unwired: 1 in, 1 out]
                      n310 = Or(x=w576, y=w575) -> (x .or. y?=w574:bool)
                      n311 = Build Array(w568, w562, w561, w560, w556, w559) -> (w558:dbl[])
                      n312 = node-c288() -> ()  [unwired: 1 in, 1 out]
                      n313 = call "LiveDataUpload.vi"("Input Array"=w558, "API String"="API Key") -> ()  [unwired: 10 in]
                    }
                  }
                }
                n314 = node-c288() -> ()  [unwired: 1 in, 1 out]
                n315 = node-c288() -> ()  [unwired: 1 in, 1 out]
              }
              n316 = local read "Hold Time\n[min]"() -> (w246:dbl)
              n317 = Multiply(x=w246, y=60000.0) -> (x*y=w245:dbl)
              n318 = Subtract(x=w245, y=12000.0) -> (x-y=w243:dbl)
              n319 = Divide(x=w243, y="t_read [ms]") -> (x/y=w239:dbl)
              n320 = Round To Nearest(number=w239) -> (nearest integer value=w238:dbl)
              n321 = Subtract(x=w238, y=2.0) -> (x-y=w233:dbl)
              "read_cnt_true" <- w233
              n322 = local read "Hold Time\n[min]"() -> (w235:dbl)
              n323 = local read "t_read [ms]"() -> (w234:dbl)
              n324 = xnode "Formula"("X1"=w235, "X2"=w233, "X3"=w234) -> ("Result"=→"t_diff":dbl)  [unwired: 1 in, 1 out]
              n325 = call <extravilib>:"Read.vi"("channel"=w242) -> ("element"=w249:bool)  [unwired: 1 in, 1 out]
              n326 = Equal?(x=w241, y=0.0) -> (x = y?=w250:bool)
              n327 = Or(x=w250, y=w249) -> (x .or. y?=w248:bool)
              n328 = node-c288(w253) -> ()  [unwired: 1 out]
            }
            n329 = node-c288() -> ()  [unwired: 1 in, 1 out]
          }
        }
      }
      n330 = node-c288() -> ()  [unwired: 1 in, 1 out]
      n331 = node-c288() -> ()  [unwired: 1 in, 1 out]
    }
    n332 = Unbundle("COM Port Settings") -> ("Baud Rate"=w37:T10, "VISA Sesssion In"=w36:refnum<visa-resource-name>)
    n333 = Bundle(cluster=T4 {"Unit ID"="A", "Baud Rate"=enum."19200", "VISA Sesssion In"="COM1"} ("Communication Settings"), "Baud Rate"=w37, "VISA Sesssion In"=w36) -> (w35:T4)  [unwired: 1 in]
    n334 = call "COM Port Initialization.vi"("error in (no error)"=errorcluster {"status"=FALSE, "code"=0, "source"=""}, "Communication Settings"=w35) -> ("error out"=w28:errorcluster, "VISA Session Out"=w27:refnum<visa-resource-name>)  [unwired: 8 in]
    n335 = Cluster To Array(cluster="Device ID's \nto Include:") -> (array=w31:bool[])
    n336 = for {
      N: 6 -> [_]
      tunnel: "ABCDEF" -> [w618]
      tunnel: w31 -> [w611] mode=indexing
      shift-right: [w610] -> _
      shift-left: u16 0 ("length (rest)") -> [w616]
      shift-right: [w615] -> w25
      shift-left: cluster{string, u16}[] [] -> [w614]
      tunnel: w28 -> [w609]
      tunnel: w27 -> [w608]
      tunnel: [w609] -> w18
      tunnel: [w608] -> w26
      i -> [w617]
      # "Generate array of Device ID's, with sequential ID's"
      n337 = Equal?(x=w611, y=TRUE) -> (x = y?=w613:bool)
      n338 = case shown="True" w613 {
        tunnel: w618 -> [_ w629]
        tunnel: w617 -> [_ w628]
        tunnel: w616 -> [w619 w621]
        tunnel: [w620 w624] -> w615
        tunnel: w614 -> [w620 w622]
        tunnel: [w619 w625] -> w610
        frame False {
          # "ID was not included"
        }
        frame True {
          # "ID was included"
          n339 = String Subset(string=w629, offset (0)=w628, length (rest)=1 ("length (rest)")) -> (substring=w626:string)
          n340 = Bundle(w626, "length (rest)"=w621) -> (w623:cluster{string, "length (rest)":u16})  [unwired: 1 in]
          n341 = Increment(x=w621) -> (x+1=w625:u16)
          n342 = Build Array (concatenate)(w622, w623) -> (w624:cluster{string, "length (rest)":u16}[])
        }
      }
    }
    n343 = property on="Active Device" class="Ring (strict)"(error in=w18, "StringsAndValues[]"=w25) -> (error out=w17:errorcluster)  [unwired: 1 in, 1 out]
    n344 = for {
      tunnel: w26 -> [w606]
      tunnel: [w603] -> w22
      tunnel: w17 -> [w607]
      tunnel: [w602] -> w21
      tunnel: w25 -> [w604] mode=indexing
      tunnel: [w605] -> w24 mode=indexing
      tunnel: [w595] -> w23 mode=indexing
      tunnel: [w601] -> w20 mode=indexing
      tunnel: [nan ("Setpoint")] -> w19 mode=indexing
      tunnel: [w594] -> w16 mode=indexing
      # "Get measurement formats, unit ID's and the controller info"
      n345 = Unbundle(w604) -> (w595:string)  [unwired: 1 out]
      n346 = property on="Active Device" class="Ring (strict)" props=["Value"]() -> ()  [unwired: 2 in, 3 out]
      n347 = call "Read Measurement Format.vi"("Unit ID (A)"=w595, "error in"=w607, "VISA Session In"=w606) -> ("error out"=w598:errorcluster, "Data Frame Format"=w605:T11, "VISA Session Out"=w599:refnum<visa-resource-name>)  [unwired: 6 in]
      n348 = call "Read Software Version.vi"("Unit ID (A)"=w595, "error in"=w598, "VISA Session In"=w599) -> ("error out"=w597:errorcluster, "Software Version"=w594:u8, "VISA Session Out"=w596:refnum<visa-resource-name>)  [unwired: 6 in]
      n349 = call "Read Controller Info.vi"("Unit ID (A)"=w595, "error in"=w597, "Software Version"=w594, "VISA Session In"=w596) -> ("error out"=w602:errorcluster, "Controller Info out"=w601:T12, "VISA Session Out"=w603:refnum<visa-resource-name>)  [unwired: 4 in, 1 out]
    }
    n350 = while {
      shift-right: [w666] -> _
      shift-left: 0.0 ("Set Start Time (s)") -> [w669]
      shift-right: [w652] -> w40
      shift-left: w21 -> [w668]
      shift-right: [w633] -> w41
      shift-left: w22 -> [w667]
      tunnel: w23 -> [w631]
      shift-right: [w654] -> _
      shift-left: w24 -> [w661]
      shift-right: [w651] -> _
      shift-left: w20 -> [w649]
      shift-right: [w647] -> _
      shift-left: w19 -> [w646]
      shift-right: [w642] -> _
      shift-left: w16 -> [w642]
      tunnel: w12 -> [w640]
      stop <- w641 stop-if-true
      # "Acquire data for every device ID included at the requested data rate, then display only the selected device's data"
      n351 = call "Elapsed Time"("Set Start Time (s)"=w669) -> ("Get Start Time (s)"=w666:dbl, "Elapsed Time (s)"=w663:dbl)  [unwired: 11 in, 6 out]
      n352 = for {
        shift-right: [w698] -> w660
        shift-left: w668 -> [w701]
        shift-right: [w699] -> w659
        shift-left: w667 -> [w700]
        tunnel: w661 -> [w695] mode=indexing
        tunnel: w631 -> [w694] mode=indexing
        tunnel: [w693] -> w658 mode=indexing
        tunnel: [w692] -> w657 mode=indexing
        tunnel: [w691] -> w656 mode=indexing
        tunnel: [w690] -> w655 mode=indexing
        tunnel: [w689] -> w654 mode=indexing
        # "Acquire data for each device"
        n353 = call "Read Measurements.vi"("error in"=w701, "Data Frame Format In"=w695, "Unit ID (A)"=w694, "VISA Session In"=w700) -> ("error out"=w698:errorcluster, "Data Frame Format Out"=w689:T11, "Data Cluster"=w692:T3, "VISA Session Out"=w699:refnum<visa-resource-name>, "Unknown Dataframe Info"=w697:bool, "Error/Overrange/Unknown String"=w691:string, "Error Present"=w696:bool, "Range Exceeded"=w690:bool)
        n354 = Or(x=w697, y=w696) -> (x .or. y?=w693:bool)
      }
      n355 = local read "Z"() -> (w637:dbl[])
      n356 = Index Array(array=w637, index=1 ("index (row)")) -> (element=w635:dbl)
      "Active Device" <- w635
      n357 = To Long Integer(number=w635) -> (32bit integer=w644:i32)
      n358 = Multiply(x=1000.0 ("y"), y=w663) -> (x*y=→"Elapsed Time [ms]\n(all units)":dbl)
      n359 = Reciprocal(x=w663) -> ()  [unwired: 1 out]
      n360 = Wait (ms)(milliseconds to wait="Minimum time between \nreadings [ms] (all units)") -> ()  [unwired: 1 out]
      n361 = for {
        tunnel: w660 -> [w672]
        tunnel: [w671] -> w653
        tunnel: w659 -> [w673]
        tunnel: [w670] -> w632
        tunnel: w658 -> [w678] mode=indexing
        tunnel: w644 -> [w680]
        tunnel: w657 -> [w677] mode=indexing
        tunnel: w656 -> [w676] mode=indexing
        tunnel: w655 -> [w675] mode=indexing
        i -> [w679]
        # "Iterate over all sets of data, only display the one selected"
        n362 = Equal?(x=w680, y=w679) -> (x = y?=w674:bool)
        n363 = case shown="True" w674 {
          tunnel: w678 -> [_ w688]
          tunnel: w677 -> [_ w683]
          tunnel: w676 -> [_ w687]
          tunnel: w675 -> [_ w686]
          tunnel: w673 -> [w682 w684]
          tunnel: w672 -> [w681 w685]
          tunnel: [w681 w685] -> w671
          tunnel: [w682 w684] -> w670
          frame False {
            # "Do nothing"
          }
          frame True {
            # "Display data"
            "Range Exceeded" <- w686
            "Error Present" <- w688
            "Error Text" <- w687
            "Meas. Data (for active device)" <- w683
          }
        }
      }
      n364 = local read "Z"() -> (w639:dbl[])
      n365 = Index Array(array=w642, index=w644) -> (element=w643:u8)
      n366 = Index Array(array=w646, index=w644) -> (element=w634:dbl)
      n367 = Index Array(array=w639, index=0) -> (element=w630:dbl)
      n368 = Replace Array Subset(array=w646, new element=w630, index=w644) -> (w647:dbl[])
      n369 = Index Array(array=w631, index=w644) -> (element=w645:string)
      n370 = Index Array(array=w649, index=w644) -> (element=w648:T12)
      n371 = call "Write SetPoint_no prev.vi"("Setpoint"=w630, "Previous Setpoint"=w634, "Unit ID (A)"=w645, "error in"=w653, "Software Version"=w643, "Controller Info out"=w648, "VISA Session In"=w632) -> ("error out"=w652:errorcluster, "Controller Info out"=w650:T12, "VISA Session Out"=w633:refnum<visa-resource-name>)  [unwired: 1 in, 1 out]
      n372 = Replace Array Subset(array=w649, new element=w650, index=w644) -> (w651:T13)
      n373 = call <extravilib>:"Read.vi"("channel"=w640) -> ("element"=w641:bool)  [unwired: 1 in, 1 out]
    }
    n374 = while "Hold Setpoints" {
      tunnel: w12 -> [w53]
      stop <- w54 stop-if-true
      n375 = call-poly <vilib>:"Read Delimited Spreadsheet.vi"("file path (dialog if empty)"="Read File", "start of read offset (chars.:0)"=0, "delimiter (\\t)"="," ("delimiter (\\t)")) -> ("all rows"=w49:dbl[][])  [unwired: 7 in, 5 out]
      "all rows" <- w49
      n376 = Array Subset(array=w49, index (row)="Start From:") -> (w47:dbl[][])  [unwired: 3 in]
      "Setpoints" <- w47
      n377 = Array Size(array=w47) -> (size(s)=w56:i32[])
      n378 = Index Array(array=w56, index=0) -> (element=→"len_SP":i32)
      n379 = call <extravilib>:"Read.vi"("channel"=w53) -> ("element"=w54:bool)  [unwired: 1 in, 1 out]
    }
    n380 = VISA Close(VISA resource name=w41, error in (no error)=w40) -> (error out=w42:errorcluster)
    n381 = Initialize Array(0.0 ("element"), 2 ("dimension size")) -> (→"Z":dbl[])
    n382 = call <vilib>:"Simple Error Handler.vi"("error in (no error)"=w42) -> ("error?"=w4:bool)  [unwired: 4 in, 4 out]
    n383 = call "CalibrationAlerts.vi"("Alert Type (0)"=5, "Trigger"=w4) -> ()  [unwired: 10 in]
    n384 = call-poly <vilib>:"Write Delimited Spreadsheet.vi"("file path (dialog if empty)"="Write File", "1D data"=string[] ["Date/Time", "Time [hh:mm:ss]", "Device ID", "P_MFC [psia]", "T_MFC [C]", "Volume Flow [LPM]", "Mass Flow [SLPM]", "SP_MFC [LPM]", "T_SCh [C]", "Iter_#", "V_D [V]", "V_H [V]", "Iter_Duration [ms]", "C_SP_CH4 [ppm]", "C_SP_H2S [ppm]"], "append to file? (new file:F)"=TRUE, "delimiter (\\t)"="," ("delimiter (\\t)")) -> ()  [unwired: 10 in, 2 out]
    n385 = node-c288(w45) -> ()  [unwired: 1 out]
  }
